vi "Delete.vi"(8 "error in (no error)":errorcluster, 11 "Config":T1) -> (0 "error out":errorcluster, 1 "Modified?":bool, 2 "Text":string, 3 "Path":path)   [LabVIEW 2022 SP3, in "LabVIEW-Config.lvlib"]
uses:
  LabVIEW-Config.lvlib
  Config.ctl
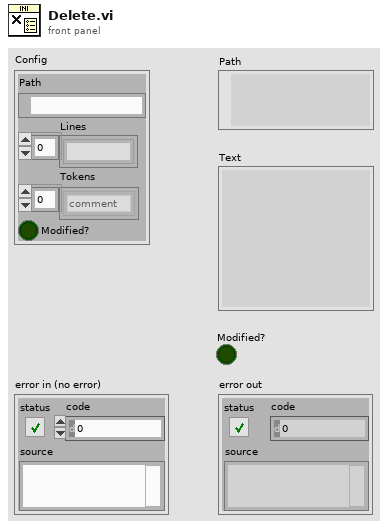
[diagram p1: front panel]
types:
  T1 = typedef "LabVIEW-Config.lvlib/Config.ctl" = cluster{"Path":path, "Lines":string[], "Tokens":enum8{"comment", "section", "key"}[], "Modified?":bool}
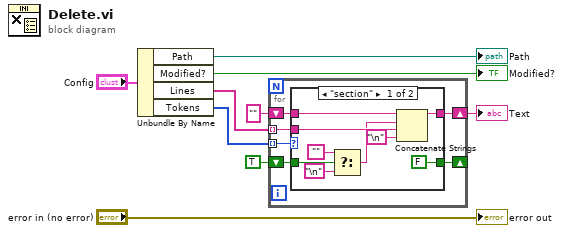
[diagram p0: block diagram]
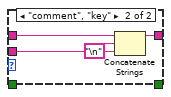
[diagram p2: hidden frame]
diagram:
  n1 = Unbundle By Name("Config") -> ("Path"=→"Path":path, "Modified?"=→"Modified?":bool, "Lines"=w7:string[], "Tokens"=w6:enum8{"comment", "section", "key"}[])
  n2 = for {
    tunnel: w7 -> [w13] mode=indexing
    tunnel: w6 -> [w15] mode=indexing
    shift-right: [w14] -> w1
    shift-left: "" -> [w12]
    shift-right: [w10] -> _
    shift-left: TRUE -> [w11]
    n3 = case shown="\"section\"" w15 {
      tunnel: [w23 w27] -> w14
      tunnel: w13 -> [w24 w28]
      tunnel: w12 -> [w21 w25]
      tunnel: w11 -> [w19 _]
      tunnel: [FALSE _] -> w10
      frame "section" {
        n4 = Select(t="" ("Empty String Constant"), s=w19, f="\n" ("Line Feed Constant")) -> (s? t:f=w17:string)
        n5 = Concatenate Strings(w21, w17, w24, "\n" ("Line Feed Constant")) -> (w23:string)
      }
      frame "comment", "key" {
        n6 = Concatenate Strings(w25, w28, "\n" ("Line Feed Constant")) -> (w27:string)
      }
    }
  }
  "Text" <- w1
  "error out" <- "error in (no error)"
